vi "Release Priority Queue.vi"(8 "error in (no error)":errorcluster, 11 "Priority Queue":refnum<class "Message Priority Queue.lvclass">) -> (0 "error out":errorcluster, 2 "remaining elements":refnum<class "Message.lvclass">[](array[class]))   [LabVIEW 2017, in "Actor Framework.lvlib" / "Message Priority Queue.lvclass"]
uses:
  <vilib>/ActorFramework/Message Priority Queue/Message Priority Queue.lvclass
  <vilib>/ActorFramework/Message/Message.lvclass
  <vilib>/ActorFramework/Message Priority Queue/Message Priority Queue.lvclass/Message Priority Queue.ctl
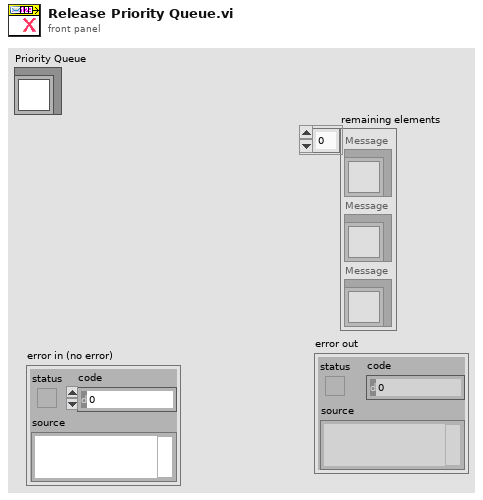
[diagram p1: front panel]
types:
  T1 = typedef "Actor Framework.lvlib/Message Priority Queue.lvclass/DVR Contents.ctl" = cluster{"# Waiting":u32, "Buffers":refnum<queue>[], "Wait Msg":refnum<queue>, "Wait Prior":refnum<queue>}
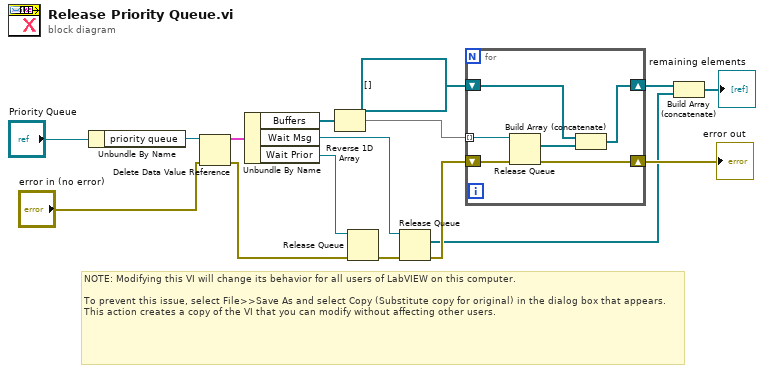
[diagram p0: block diagram]
diagram:
  # "NOTE: Modifying this VI will change its behavior for all users of LabVIEW on this computer.\n\nTo prevent this issue, select File>>Save As and select Copy (Substitute copy for original) in the dialog box that appears. This action creates a copy of the VI that you can modify without affecting other users."
  n1 = Unbundle By Name("Priority Queue") -> ("priority queue"=w12:refnum<data-value>)
  n2 = Delete Data Value Reference(data value reference=w12, error in="error in (no error)") -> (data value=w15:T1, error out=w7:errorcluster)
  n3 = Unbundle By Name(w15) -> ("Buffers"=w16:refnum<queue>[], "Wait Msg"=w3:refnum<queue>, "Wait Prior"=w1:refnum<queue>)
  n4 = Reverse 1D Array(array=w16) -> (reversed array=w10:refnum<queue>[])
  n5 = Release Queue(queue=w1, error in (no error)=w7) -> (error out=w5:errorcluster)  [unwired: 1 in, 2 out]
  n6 = Release Queue(queue=w3, error in (no error)=w5) -> (remaining elements=w2:refnum<class "Message.lvclass">[], error out=w4:errorcluster)  [unwired: 1 in, 1 out]
  n7 = for {
    tunnel: w10 -> [w22] mode=indexing
    shift-right: [w20] -> w9
    shift-left: refnum<class "Message.lvclass">[] [] -> [w19]
    shift-right: [w17] -> w8
    shift-left: w4 -> [w18]
    n8 = Release Queue(queue=w22, error in (no error)=w18) -> (remaining elements=w21:refnum<class "Message.lvclass">[], error out=w17:errorcluster)  [unwired: 1 in, 1 out]
    n9 = Build Array (concatenate)(w19, w21) -> (w20:refnum<class "Message.lvclass">[])
  }
  "error out" <- w8
  n10 = Build Array (concatenate)(w9, w2) -> (→"remaining elements":refnum<class "Message.lvclass">[])
